vi "Process.vi"(8 "error in":errorcluster, 11 "Example Instrument UI":refnum<class "Instrument UI.Framework-Template.lvclass">) -> (0 "error out":errorcluster, 3 "Example Instrument UI out":refnum<class "Instrument UI.Framework-Template.lvclass">)   [LabVIEW 2019, in "Instrument UI.Framework-Template.lvclass"]
doc: "---------------------------------------------------------------\nJKI State Machine Objects™\nhttp://jki.net/state-machine-objects/\nCopyright (C) 2005-2015, JKI <info@jki.net>\nALL RIGHTS RESERVEDJKI State Machine Objects (SMO) 1.0.0.5\nJKI - JKI\nCopyright (c) 2016, JKI"
uses:
  Instrument UI.Framework-Template.lvclass
  C:/Program Files (x86)/National Instruments/LabVIEW 2019/vi.lib/JKI/JKI SMO/SMO/SMO.lvclass
  C:/Users/patrick/Documents/GitHub/Instrument-Framework/lvsrc/SMOs/Instrument UI/Instrument UI.lvclass
  C:/Program Files (x86)/National Instruments/LabVIEW 2019/vi.lib/JKI/JKI SMO/SMO.UI/SMO.UI.lvclass
  Instrument.Framework-Template/Typedefs/Instrument.Framework-Template.getAll--Cluster.ctl
  Instrument.Framework-Template/Instrument.Framework-Template.lvclass
  C:/Users/patrick/Documents/GitHub/Instrument-Framework/lvsrc/SMOs/Instrument/Instrument.lvclass
  Instrument UI.Framework-Template.UI--Cluster.ctl
  Instrument.Framework-Template/Typedefs/Instrument.Framework-Template.Configuration--Cluster.ctl
  SMOs/Configuration/Configuration.lvclass
  SMOs/Instrument UI/Instrument UI.lvclass/Instrument UI.ctl
  <vilib>/JKI/JKI SMO/SMO/SMO.lvclass/SMO.ctl
  SMOs/Configuration/Configuration.lvclass/Configuration.ctl
  SMOs/Instrument/Instrument.lvclass/Instrument.ctl
  SMOs/Instrument/Typedefs/Client Type--Enum.ctl
  614f1787-3484-4d72-b522-1f8c221dac07.vi
  064e3a37-d4cf-416d-9c97-81a00de9d50c.vi
  <vilib>/JKI/JKI SMO/SMO/Private/ReftoDVR--SMO.vi
  614f1787-3484-4d72-b522-1f8c221dac07.vi/6126265b-52a9-4036-b9ab-d7def26448fd.vi
  064e3a37-d4cf-416d-9c97-81a00de9d50c.vi/2934c5b6-9d9a-4612-aef0-474eff5135e3.vi
  614f1787-3484-4d72-b522-1f8c221dac07.vi/6126265b-52a9-4036-b9ab-d7def26448fd.vi/3777206e-62d3-4194-bbb6-d708f28c6636.vi
  SMOs/Instrument/API/Send and Receive.vi
  614f1787-3484-4d72-b522-1f8c221dac07.vi/6126265b-52a9-4036-b9ab-d7def26448fd.vi/c2acc09a-a3b2-411f-96f0-93bdcc04d904.vi
  SMOs/Instrument/Private/Get Client Type.vi
  064e3a37-d4cf-416d-9c97-81a00de9d50c.vi/2934c5b6-9d9a-4612-aef0-474eff5135e3.vi/d31bd197-f2cf-45ec-b348-66ecc1fb7fa3.vi
  064e3a37-d4cf-416d-9c97-81a00de9d50c.vi/2934c5b6-9d9a-4612-aef0-474eff5135e3.vi/bcf0d896-5092-4459-a902-822cb84f3d2f.vi
  614f1787-3484-4d72-b522-1f8c221dac07.vi/6126265b-52a9-4036-b9ab-d7def26448fd.vi/3777206e-62d3-4194-bbb6-d708f28c6636.vi/a171245e-ace2-4a31-ad0e-c1ba96aac09f.vi
  614f1787-3484-4d72-b522-1f8c221dac07.vi/6126265b-52a9-4036-b9ab-d7def26448fd.vi/3777206e-62d3-4194-bbb6-d708f28c6636.vi/314606e5-fab2-4c4b-855f-38e561406072.vi
  614f1787-3484-4d72-b522-1f8c221dac07.vi/6126265b-52a9-4036-b9ab-d7def26448fd.vi/c2acc09a-a3b2-411f-96f0-93bdcc04d904.vi/068c89fb-261c-4114-b3e0-8879b2039521.vi
  614f1787-3484-4d72-b522-1f8c221dac07.vi/6126265b-52a9-4036-b9ab-d7def26448fd.vi/c2acc09a-a3b2-411f-96f0-93bdcc04d904.vi/70e8e4d8-081c-4447-abab-7ffc08a24431.vi
  064e3a37-d4cf-416d-9c97-81a00de9d50c.vi/2934c5b6-9d9a-4612-aef0-474eff5135e3.vi/d31bd197-f2cf-45ec-b348-66ecc1fb7fa3.vi/16df6886-ccac-4f12-823d-852507d7b6d3.vi
  064e3a37-d4cf-416d-9c97-81a00de9d50c.vi/2934c5b6-9d9a-4612-aef0-474eff5135e3.vi/d31bd197-f2cf-45ec-b348-66ecc1fb7fa3.vi/d363edf0-f48d-4095-b52d-a98fc5c23e31.vi
  064e3a37-d4cf-416d-9c97-81a00de9d50c.vi/2934c5b6-9d9a-4612-aef0-474eff5135e3.vi/bcf0d896-5092-4459-a902-822cb84f3d2f.vi/3efd9854-12da-426d-b303-5f5dfdd99cd3.vi
  064e3a37-d4cf-416d-9c97-81a00de9d50c.vi/2934c5b6-9d9a-4612-aef0-474eff5135e3.vi/bcf0d896-5092-4459-a902-822cb84f3d2f.vi/021688bb-175a-4f04-92c2-7b75fc3f16e3.vi
  614f1787-3484-4d72-b522-1f8c221dac07.vi/6126265b-52a9-4036-b9ab-d7def26448fd.vi/c2acc09a-a3b2-411f-96f0-93bdcc04d904.vi/068c89fb-261c-4114-b3e0-8879b2039521.vi/f4340ad4-3f7d-43fc-a5b8-8cfecf0320e0.vi
  614f1787-3484-4d72-b522-1f8c221dac07.vi/6126265b-52a9-4036-b9ab-d7def26448fd.vi/c2acc09a-a3b2-411f-96f0-93bdcc04d904.vi/068c89fb-261c-4114-b3e0-8879b2039521.vi/09137493-ac28-451c-9813-f227a1b20a03.vi
  064e3a37-d4cf-416d-9c97-81a00de9d50c.vi/2934c5b6-9d9a-4612-aef0-474eff5135e3.vi/bcf0d896-5092-4459-a902-822cb84f3d2f.vi/3efd9854-12da-426d-b303-5f5dfdd99cd3.vi/ec8d0cc2-9f9f-4698-9277-550a01addf9f.vi
  064e3a37-d4cf-416d-9c97-81a00de9d50c.vi/2934c5b6-9d9a-4612-aef0-474eff5135e3.vi/bcf0d896-5092-4459-a902-822cb84f3d2f.vi/3efd9854-12da-426d-b303-5f5dfdd99cd3.vi/599ad89e-f603-4806-a637-659fe558540e.vi
  SMOs/Instrument/Private/Get RC Connection Status.vi
  SMOs/Instrument/API/Enum to String.vi
  SMOs/RemoteControl/API/Send and Receive.vi
  <vilib>/Utility/Data Type/Get Type Information.vi
  <vilib>/JDP Science/JSONtext/JSON text to Variant.vi
  <vilib>/JDP Science/JSONtext/Variant to JSON Text.vi
  <vilib>/National Instruments/GUID Generator/Guid Generator.vi
  SMOs/Instrument/Private/Instrument.MessageFromProcess.EventStructure.vi
  SMOs/Instrument/Instrument.lvclass
  <vilib>/JDP Science/JSONtext/LVClass Serializer/JSONtext LVClass Serializer.lvclass
  SMOs/Instrument UI/Instrument UI.lvclass
  <vilib>/JKI/JKI SMO/SMO/SMO.lvclass
  <vilib>/JKI/JKI SMO/SMO.UI/SMO.UI.lvclass
panel:
  in  "Parameter 2":string
  out "Numeric":u32
  in  "Set Parameter":bool
  in  "Parameter":dbl
  in  "STOP":bool
  out "SMO string":string
  out "SMO Boolean":bool
  out "Logger SMO":dbl
  out "Levy 1":dbl
  # "#todo\nmake UI here. maybe include a nice picture of the hardware?"
  # "#todo\nadd buttons to do stuff (e.g., change a setting)\nButtons should trigger an event"
  # "#todo\nresize this box if you want your UI to be different size"
  # "SMO UI Template"
  # "For instructions on how to use the JKI State Machine Objects, examples and video tutorials, visit:\nhttp://jki.net/state-machine-objects/\n\nJKI State Machine Objects™\nhttp://jki.net/state-machine-objects/\nCopyright (C) 2005-2015, JKI <info@jki.net>\nALL RIGHTS RESERVED"
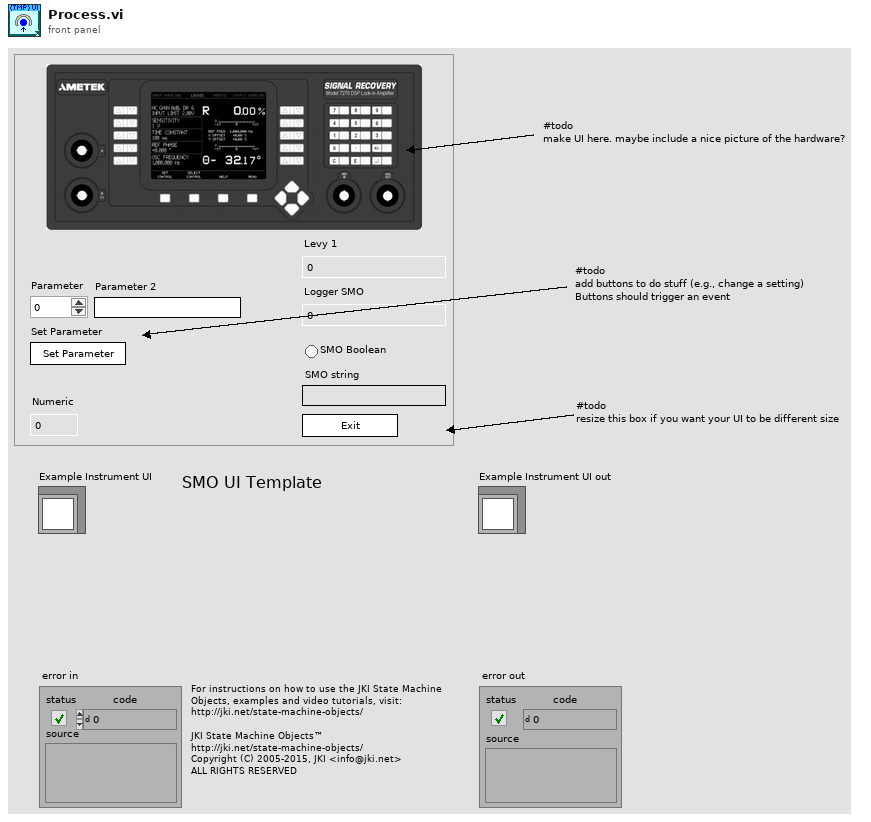
[diagram p1: front panel]
types:
  T1 = enum32{"invalid app kind", "Development System", "Run Time System", "Student Edition", "Embedded LabVIEW", "Evaluation", "Custom"}
  T2 = enum32{"Invalid", "Standard", "Closed", "Hidden", "Minimized", "Maximized"}
  T3 = typedef "Instrument.lvclass/Client Type--Enum.ctl" = enum16{"Remote", "Local"}
  T4 = typedef "Instrument.Framework-Template.lvclass/Instrument.Framework-Template.Configuration--Cluster.ctl" = cluster{"Example Setting 1":dbl, "Example Setting 2":dbl, "Example Setting 3":string}
  T5 = typedef "Instrument.Framework-Template.lvclass/Instrument.Framework-Template.getAll--Cluster.ctl" = cluster{"Levy 1":dbl, "Logger SMO":dbl, "SMO Boolean":bool, "SMO String":string}
  T6 = typedef "Instrument UI.Framework-Template.lvclass/Instrument UI.Framework-Template.UI--Cluster.ctl" = cluster{"Parameter":dbl, "Parameter 2":string}
  T7 = cluster{"Core":cluster{"Current VI Reference":refnum<vi>, "Close Panel on Exit?":bool, "error":errorcluster}, "Instrument UI":refnum<class "Instrument UI.Framework-Template.lvclass">, "Instrument":refnum<class "Instrument.Framework-Template.lvclass">, "Configuration":refnum<class "Configuration.lvclass">, "Config Cluster":T4, "getAll":T5, "UI Cluster":T6}
  T8 = cluster{"Current VI Reference":refnum<vi>, "Close Panel on Exit?":bool, "error":errorcluster}
  T9 = typedef "SMO.lvclass/Protected Events.ctl" = cluster{"StopProcesses":refnum<user-event>, "AbortProcesses":refnum<user-event>, "Config Changed":refnum<user-event>, "Dependency":refnum<user-event>}
  T10 = typedef "Instrument.lvclass/PublicEvents--Cluster.ctl" = cluster{"MessageFromProcess":refnum<user-event>}
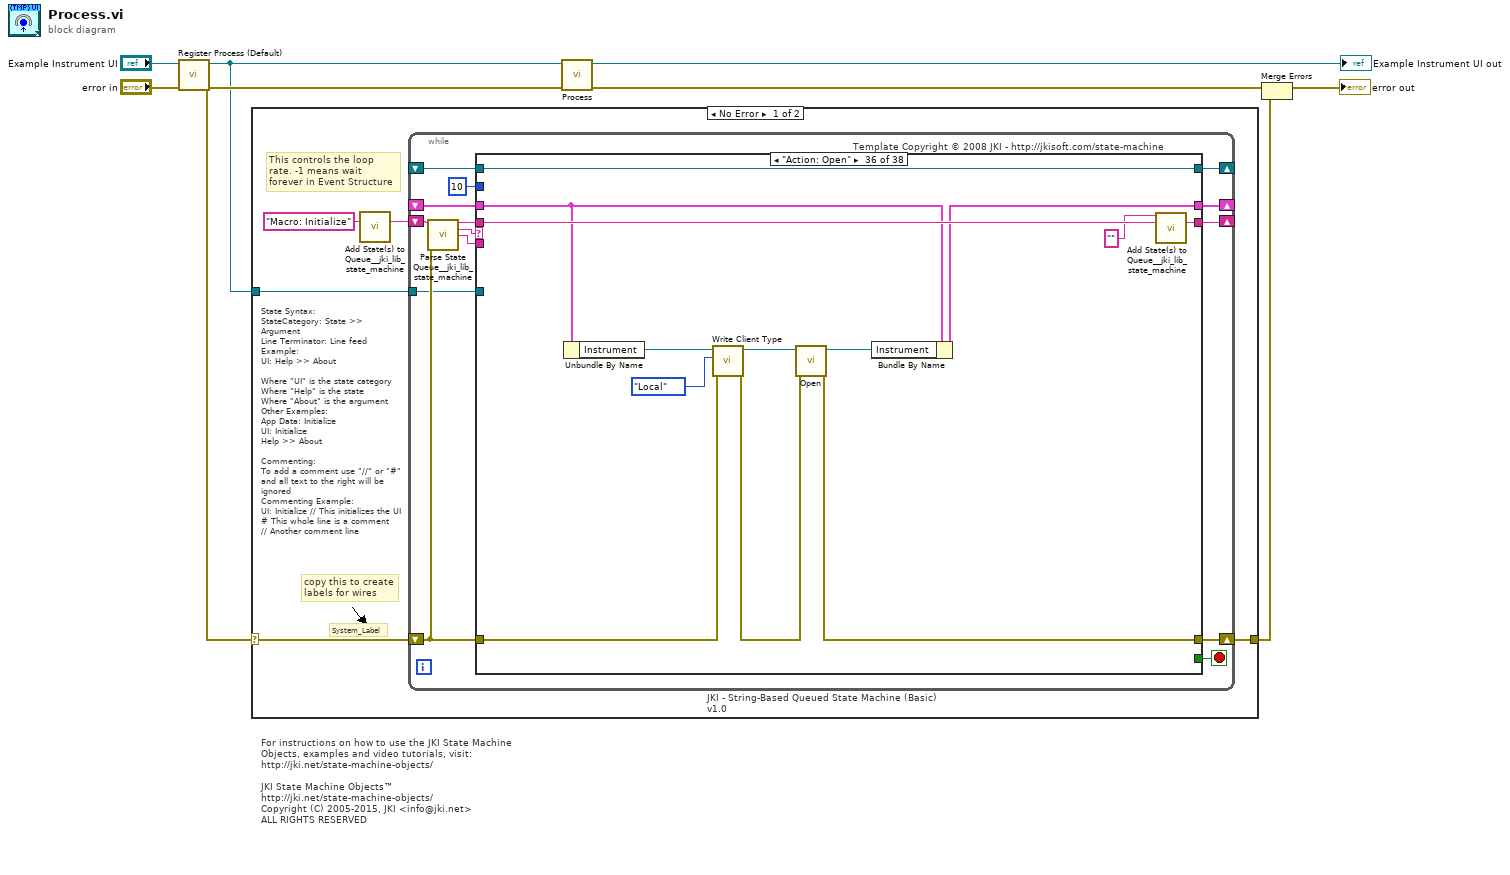
[diagram p0: block diagram]
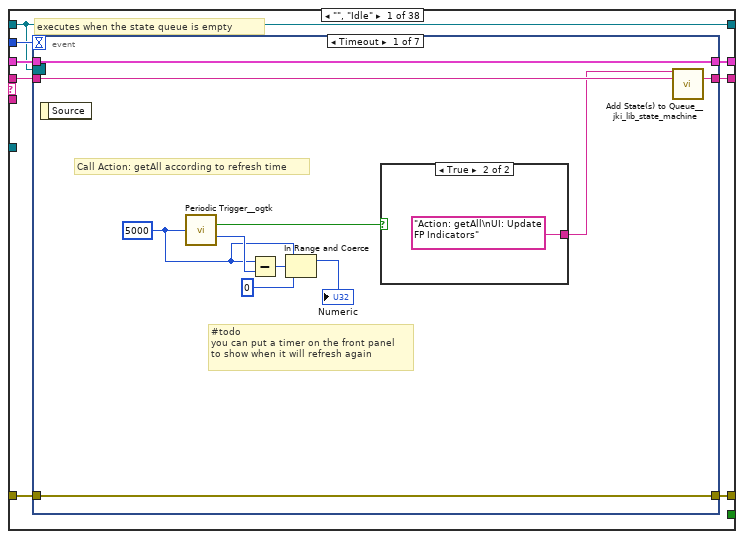
[diagram p2: hidden frame]
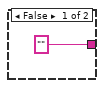
[diagram p3: hidden frame]
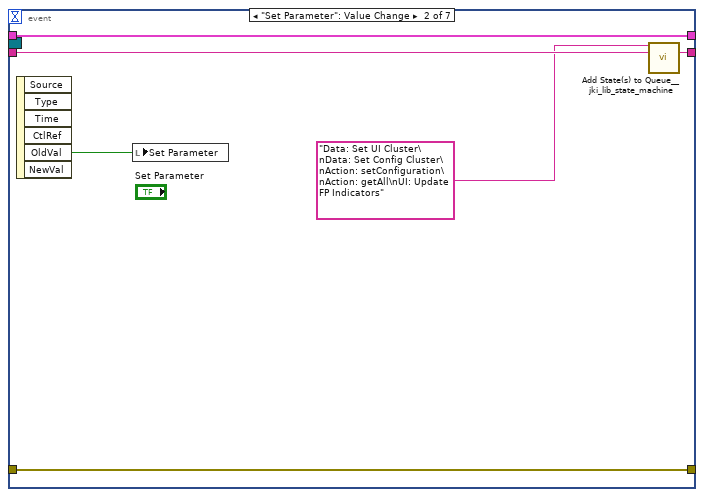
[diagram p4: hidden frame]
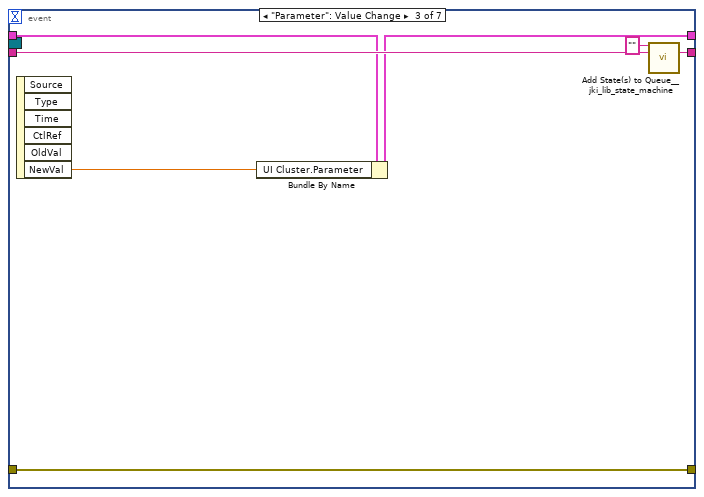
[diagram p5: hidden frame]
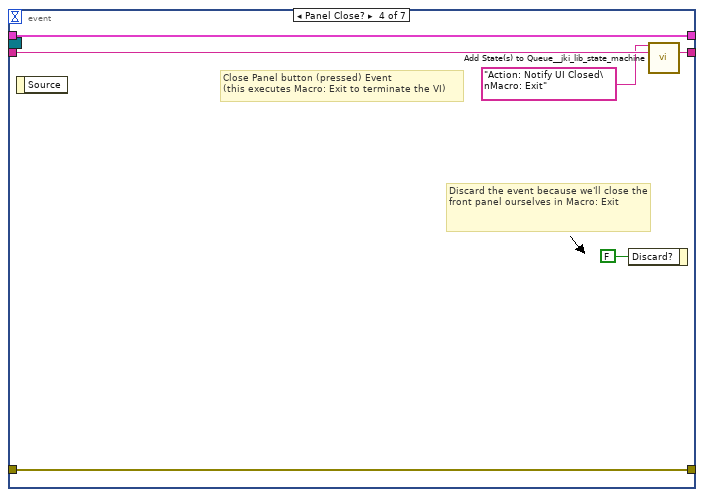
[diagram p6: hidden frame]
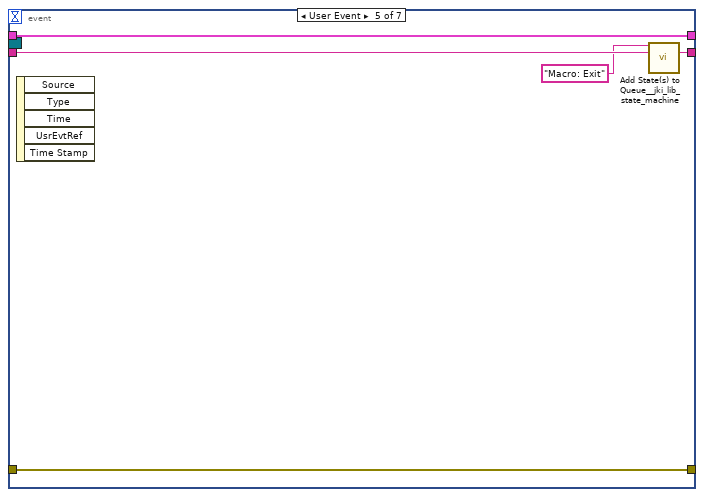
[diagram p7: hidden frame]
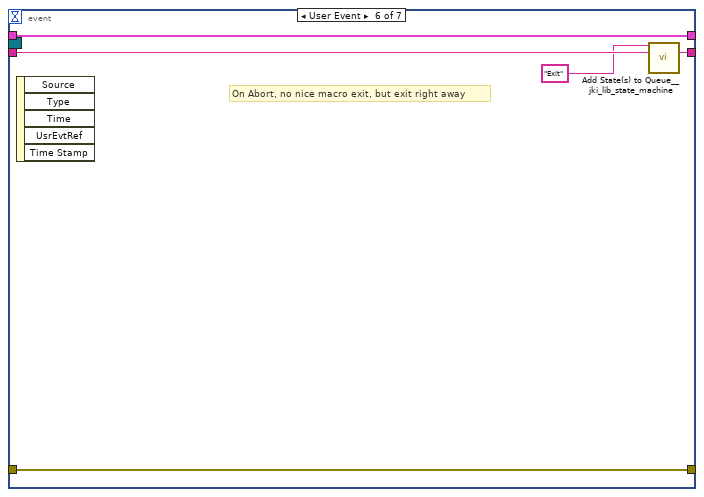
[diagram p8: hidden frame]
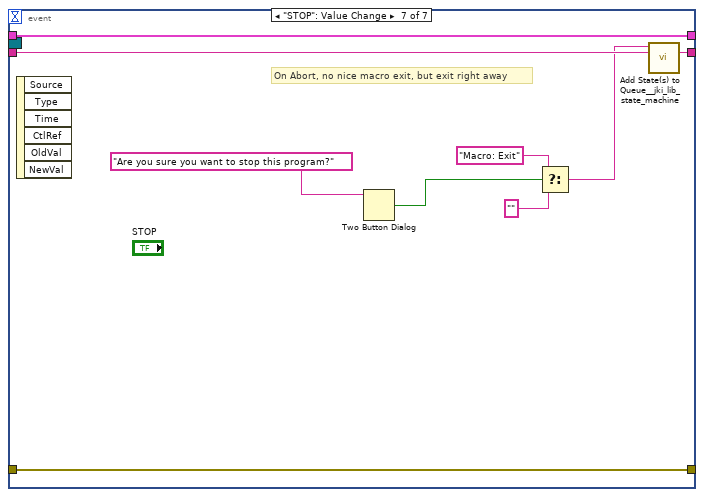
[diagram p9: hidden frame]
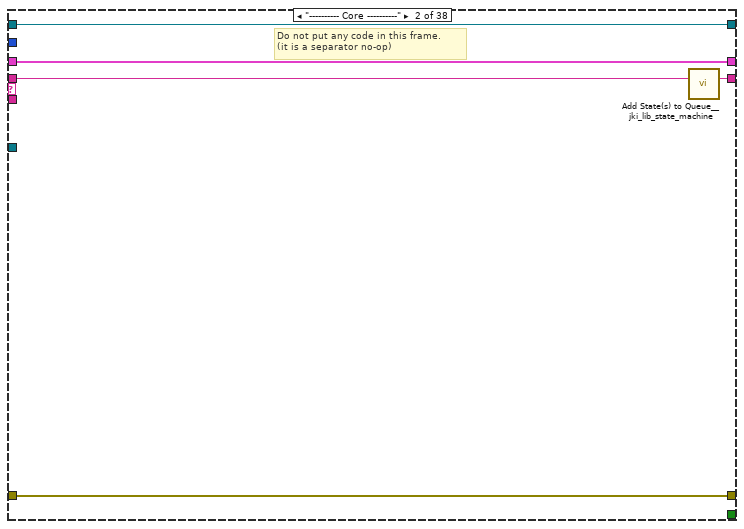
[diagram p10: hidden frame]
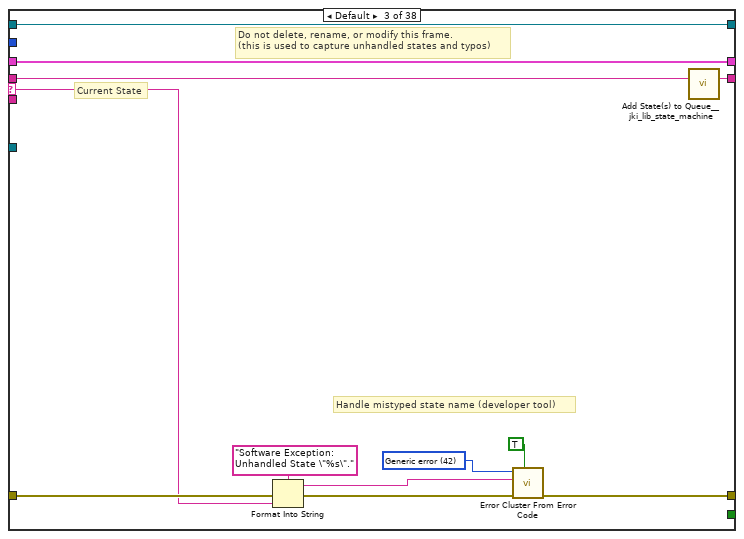
[diagram p11: hidden frame]
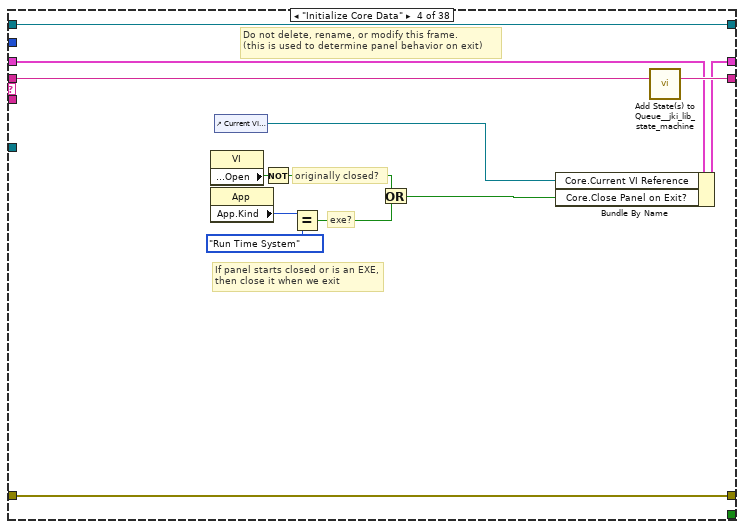
[diagram p12: hidden frame]
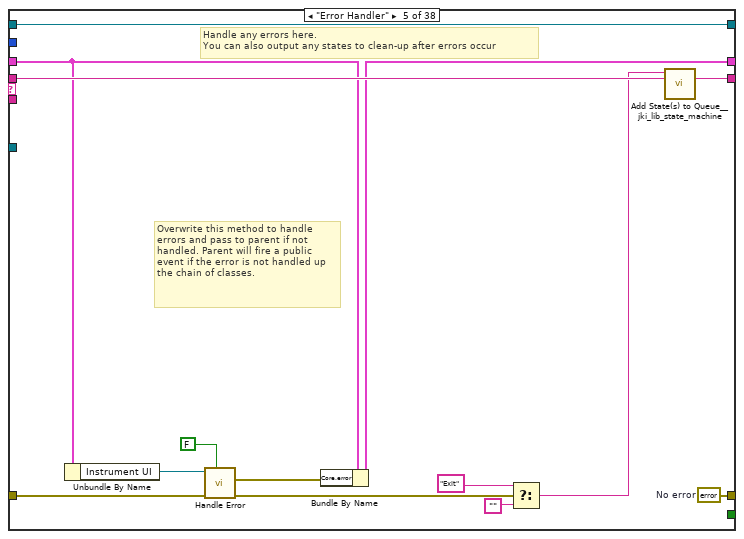
[diagram p13: hidden frame]
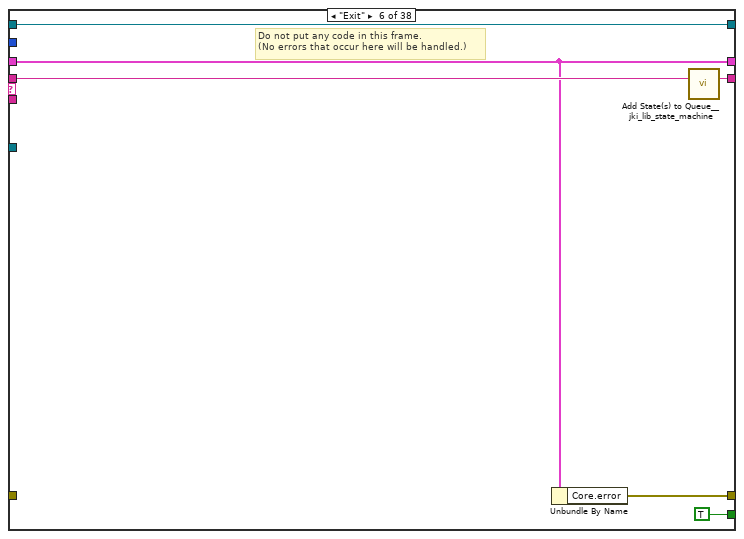
[diagram p14: hidden frame]
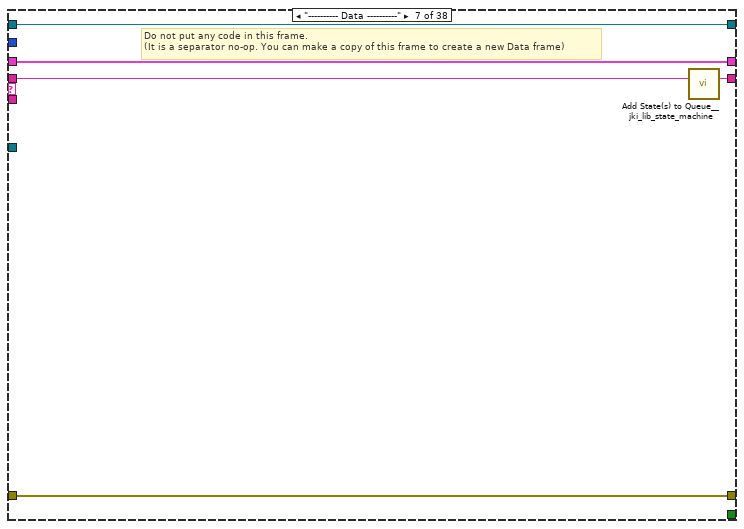
[diagram p15: hidden frame]
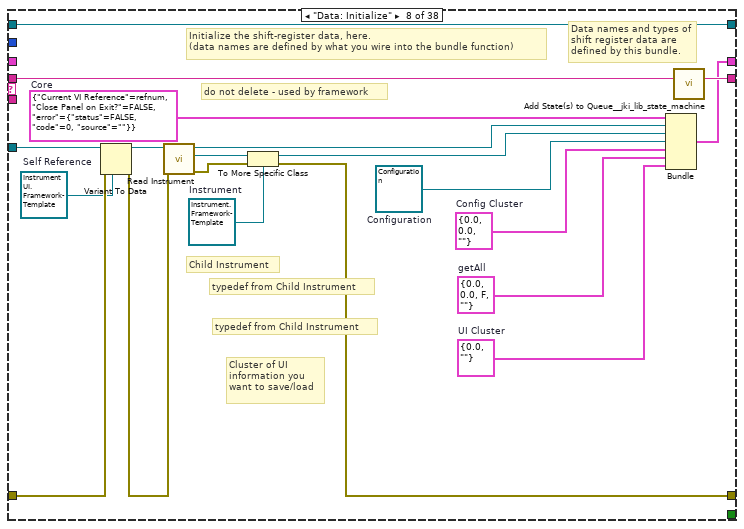
[diagram p16: hidden frame]
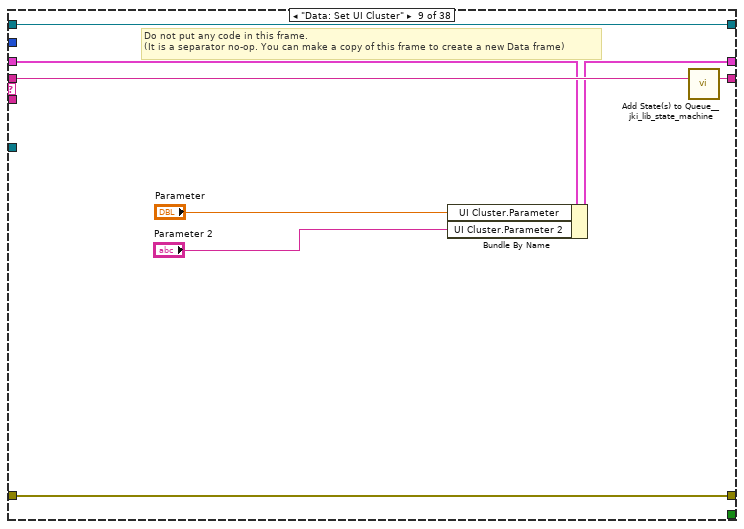
[diagram p17: hidden frame]
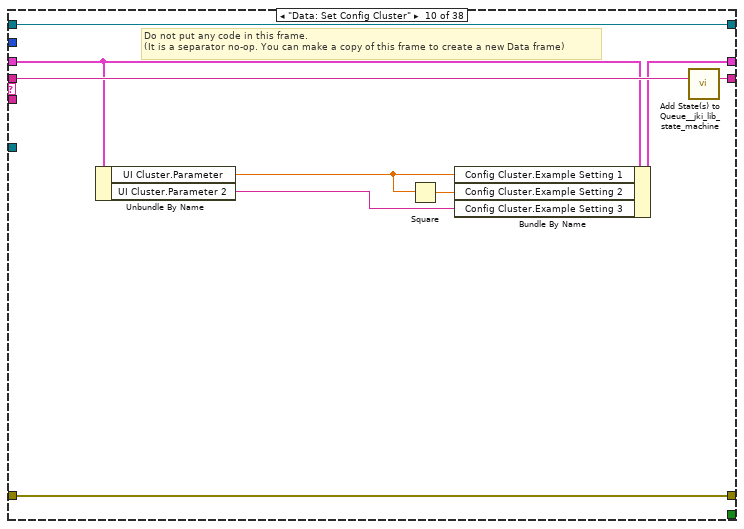
[diagram p18: hidden frame]
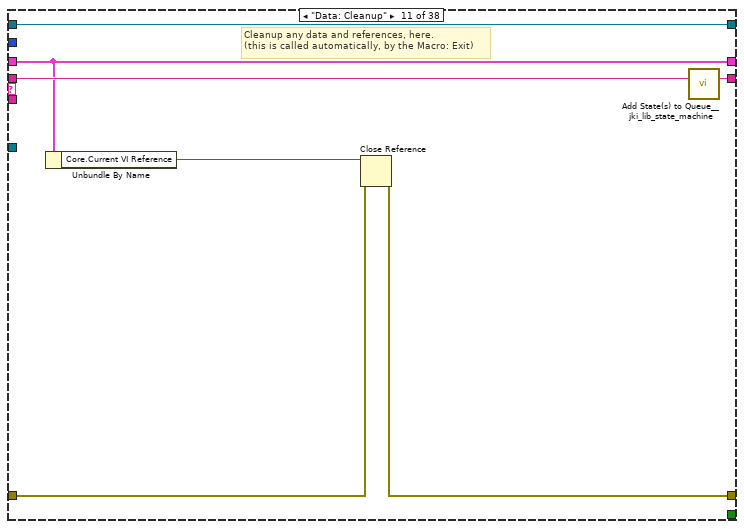
[diagram p19: hidden frame]
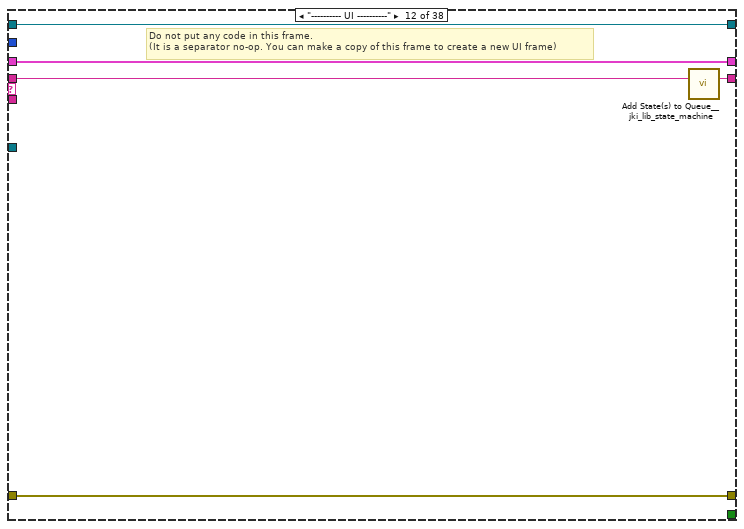
[diagram p20: hidden frame]
diagram:
  # "For instructions on how to use the JKI State Machine Objects, examples and video tutorials, visit:\nhttp://jki.net/state-machine-objects/\n\nJKI State Machine Objects™\nhttp://jki.net/state-machine-objects/\nCopyright (C) 2005-2015, JKI <info@jki.net>\nALL RIGHTS RESERVED"
  n1 = call <vilib>:"Register Process (Default).vi"("error in (no error)"="error in", "SMO"="Example Instrument UI") -> ("error out"=w5:errorcluster, "SelfRef"=w4:refnum<class "Instrument UI.Framework-Template.lvclass">)  [unwired: 8 in]
  n2 = case shown="No Error" w5 {
    selector: w5 -> [w10 w453]
    tunnel: w4 -> [w11 _]
    tunnel: [w9 w453] -> w1
    frame No Error {
      # "State Syntax:\nStateCategory: State >> Argument\nLine Terminator: Line feed\nExample:\nUI: Help >> About\n\nWhere \"UI\" is the state category\nWhere \"Help\" is the state\nWhere \"About\" is the argument\nOther Examples:\nApp Data: Initialize\nUI: Initialize\nHelp >> About\n\nCommenting:\nTo add a comment use \"//\" or \"#\" and all text to the right will be ignored\nCommenting Example:\nUI: Initialize // This initializes the UI\n# This whole line is a comment\n// Another comment line"
      # "copy this to create labels for wires"
      # "This controls the loop rate. -1 means wait forever in Event Structure"
      # "System_Label"
      n3 = call <vilib>:"Add State(s) to Queue__jki_lib_state_machine.vi"("State(s) in (\"\")"="Macro: Initialize") -> ("States Out"=w13:string)  [unwired: 14 in]
      n4 = while "JKI - String-Based Queued State Machine (Basic) v1.0" {
        shift-right: [w20] -> _
        shift-left: _ -> [w19]
        shift-right: [w23] -> w9
        shift-left: w10 -> [w17]
        shift-right: [w22] -> _
        shift-left: w13 -> [w24]
        tunnel: w11 -> [w16]
        shift-right: [w15] -> _
        shift-left: _ -> [w14]
        stop <- w21 stop-if-true
        # "Template Copyright © 2008 JKI - http://jkisoft.com/state-machine"
        n5 = call <vilib>:"Parse State Queue__jki_lib_state_machine.vi"("State Queue"=w24, "Error In (no error)"=w17) -> ("Remaining States"=w26:string, "Current State"=w27:string, "Arguments"=w25:string)  [unwired: 11 in]
        n6 = case shown="\"Action: Open\"" w27 {
          selector: w27 -> [_ _ w93 _ _ _ _ _ _ _ _ _ _ _ _ _ _ _ _ _ _ _ _ _ _ _ _ _ _ _ _ _ _ _ _ _ _ _]
          tunnel: w26 -> [w35 w91 w97 w116 w130 w136 w141 w161 w169 w178 w185 w190 w197 w204 w214 w221 w237 w269 w278 w284 w290 w305 w310 w321 w328 w333 w346 w352 w357 w372 w380 w392 w399 w406 w418 w431 w441 w452]
          tunnel: w25 -> [_ _ _ _ _ _ _ _ _ _ _ _ _ _ _ w215 w231 _ _ _ _ _ _ _ _ _ _ _ _ _ _ _ _ _ _ _ _ _]
          tunnel: w19 -> [w33 w88 w95 w107 w119 w132 w138 _ w165 w174 w179 w187 w195 w200 w205 w219 w233 w266 w274 w281 w287 w292 w307 w318 w323 w330 w344 w350 w354 w365 w377 w383 w395 w400 w410 w425 w433 w444]
          tunnel: [w32 w89 w99 w113 w121 w131 w139 w143 w167 w176 w181 w188 w192 w202 w206 w216 w234 w267 w276 w282 w288 w303 w308 w312 w324 w331 w339 w347 w355 w358 w375 w384 w396 w401 w415 w428 w438 w449] -> w23
          tunnel: w17 -> [w31 w89 w98 w113 w126 _ w139 w158 w167 w176 w182 w188 w193 w202 w206 w217 w235 w267 w276 w282 w288 w303 w308 w313 w325 w331 w341 w348 w355 w367 w373 w385 w396 w402 w411 w420 w434 w445]
          tunnel: [w34 w90 w96 w115 w129 w135 w140 w160 w168 w177 w184 w189 w196 w203 w213 w220 w236 w268 w277 w283 w289 w304 w309 w320 w327 w332 w345 w351 w356 w371 w379 w391 w398 w405 w417 w430 w440 w451] -> w22
          tunnel: [_ _ _ _ _ TRUE _ _ _ _ _ _ _ _ _ _ _ _ _ _ _ _ _ _ _ _ _ _ _ _ _ _ _ _ _ _ _ _] -> w21
          tunnel: [w30 w88 w95 w114 w118 w132 w138 w159 w164 w173 w179 w187 w195 w200 w205 w219 w233 w266 w274 w281 w287 w292 w307 w318 w323 w330 w344 w350 w354 w369 w377 w381 w394 w400 w412 w426 w435 w446] -> w20
          tunnel: 10 ("Timeout") -> [w29 _ _ _ _ _ _ _ _ _ _ _ _ _ _ _ _ _ _ _ _ _ _ _ _ _ _ _ _ _ _ _ _ _ _ _ _ _]
          tunnel: w16 -> [_ _ _ _ _ _ _ w156 _ _ _ _ _ _ _ _ _ _ _ _ _ _ _ _ _ _ _ _ _ _ _ _ _ _ _ _ _ _]
          tunnel: [w28 w87 w92 w104 w128 w133 w137 w155 w166 w175 w180 w186 w194 w201 w212 w218 w230 w265 w275 w280 w286 w297 w306 w319 w326 w329 w343 w349 w353 w370 w378 w390 w397 w404 w416 w429 w439 w450] -> w15
          tunnel: w14 -> [w28 w87 w92 w104 w128 w133 w137 w155 w166 w175 w180 w186 w194 w201 w212 w218 w230 w265 w275 w280 w286 w297 w306 w319 w326 w329 _ w349 w353 w370 w378 w390 w397 w404 w416 w429 w439 w450]
          frame "", "Idle" {
            # "executes when the state queue is empty"
            n7 = event shown="[0] Timeout" {
              selector: w28 -> [_ _ _ _ _ _ _]
              dyn-events: _ -> [_ _ _ _ _ _ _]
              timeout: w29 -> [_ _ _ _ _ _ _]
              tunnel: w35 -> [w46 w54 w61 w67 w72 w77 w86]
              tunnel: [w45 w53 w60 w66 w71 w76 w85] -> w34
              tunnel: w33 -> [w43 w51 w57 w63 w69 w74 w83]
              tunnel: [w44 w52 w59 w62 w70 w75 w84] -> w32
              tunnel: w31 -> [w44 w52 w59 w62 w70 w75 w84]
              tunnel: [w43 w51 w56 w63 w69 w74 w83] -> w30
              event Timeout {
                w37 = u32 5000 ("time (ms)")
                # "#todo\nyou can put a timer on the front panel\nto show when it will refresh again"
                # "Call Action: getAll according to refresh time"
                n8 = event-data() -> ()  [unwired: 1 in, 1 out]
                n9 = call <userlib>:"Periodic Trigger__ogtk.vi"("time (ms)"=w37) -> ("Triggered"=w41:bool, "timer value"=w40:u32)  [unwired: 12 in, 1 out]
                n10 = Subtract(x=w37, y=w40) -> (x-y=w39:u32)
                n11 = In Range and Coerce(upper limit=w37, x=w39, lower limit=u32 0) -> (coerced(x)=→"Numeric":u32)  [unwired: 1 out]
                n12 = case shown="True" w41 {
                  tunnel: ["" ("State(s) in Front (\"\")") "Action: getAll\nUI: Update FP Indicators" ("State(s) in Front (\"\")")] -> w42
                  frame False {
                  }
                  frame True {
                  }
                }
                n13 = call <vilib>:"Add State(s) to Queue__jki_lib_state_machine.vi"("State(s) in Front (\"\")"=w42, "State(s) in (\"\")"=w46) -> ("States Out"=w45:string)  [unwired: 13 in]
              }
              event "Set Parameter": Value Change {
                n14 = event-data() -> ("OldVal"=w50:bool)  [unwired: 1 in, 5 out]
                n15 = local write "Set Parameter"(w50) -> ()
                n16 = call <vilib>:"Add State(s) to Queue__jki_lib_state_machine.vi"("State(s) in Front (\"\")"="Data: Set UI Cluster\nData: Set Config Cluster\nAction: setConfiguration\nAction: getAll\nUI: Update FP Indicators" ("State(s) in Front (\"\")"), "State(s) in (\"\")"=w54) -> ("States Out"=w53:string)  [unwired: 13 in]
              }
              event "Parameter": Value Change {
                n17 = event-data() -> ("NewVal"=w58:dbl)  [unwired: 1 in, 5 out]
                n18 = Bundle By Name(cluster=w57, "UI Cluster.Parameter"=w58) -> (w56:T7)
                n19 = call <vilib>:"Add State(s) to Queue__jki_lib_state_machine.vi"("State(s) in Front (\"\")"="" ("State(s) in Front (\"\")"), "State(s) in (\"\")"=w61) -> ("States Out"=w60:string)  [unwired: 13 in]
              }
              event Panel Close? {
                # "Discard the event because we'll close the front panel ourselves in Macro: Exit"
                # "Close Panel button (pressed) Event\n(this executes Macro: Exit to terminate the VI)"
                n20 = event-data() -> ()  [unwired: 1 in, 1 out]
                n21 = event-data("Discard?"=FALSE) -> ()  [unwired: 1 in, 1 out]
                n22 = call <vilib>:"Add State(s) to Queue__jki_lib_state_machine.vi"("State(s) in Front (\"\")"="Action: Notify UI Closed\nMacro: Exit", "State(s) in (\"\")"=w67) -> ("States Out"=w66:string)  [unwired: 13 in]
              }
              event User Event {
                n23 = event-data() -> ()  [unwired: 1 in, 5 out]
                n24 = call <vilib>:"Add State(s) to Queue__jki_lib_state_machine.vi"("State(s) in Front (\"\")"="Macro: Exit", "State(s) in (\"\")"=w72) -> ("States Out"=w71:string)  [unwired: 13 in]
              }
              event User Event {
                # "On Abort, no nice macro exit, but exit right away"
                n25 = event-data() -> ()  [unwired: 1 in, 5 out]
                n26 = call <vilib>:"Add State(s) to Queue__jki_lib_state_machine.vi"("State(s) in Front (\"\")"="Exit", "State(s) in (\"\")"=w77) -> ("States Out"=w76:string)  [unwired: 13 in]
              }
              event "STOP": Value Change {
                # "On Abort, no nice macro exit, but exit right away"
                n27 = event-data() -> ()  [unwired: 1 in, 6 out]
                n28 = Two Button Dialog(message="Are you sure you want to stop this program?") -> (T button?=w82:bool)  [unwired: 2 in]
                n29 = Select(t="Macro: Exit", s=w82, f="") -> (s? t:f=w78:string)
                n30 = call <vilib>:"Add State(s) to Queue__jki_lib_state_machine.vi"("State(s) in Front (\"\")"=w78, "State(s) in (\"\")"=w86) -> ("States Out"=w85:string)  [unwired: 13 in]
              }
            }
          }
          frame "---------- Core ----------" {
            # "Do not put any code in this frame.\n(it is a separator no-op)"
            n31 = call <vilib>:"Add State(s) to Queue__jki_lib_state_machine.vi"("State(s) in (\"\")"=w91) -> ("States Out"=w90:string)  [unwired: 14 in]
          }
          frame Default {
            w102 = 42 items=["No error", "Argument error", "Memory is full", "Out of zone", "End of file", "File already open", "Generic file I/O error", "File not found", "File permission error", "Disk is full", "Duplicate path", "Too many files open", "System feature not enabled", "Resource file not found", "Cannot add resource", "Resource not found", "Image not found", "Image memory error", "Pen does not exist", "Config type invalid", "Config token not found", "Config parse error", "Config memory error", "Bad external code format", "Bad external code offset", "External code not present", "Null window", "Destroy window error", "Null menu", "Print aborted", "Bad print record", "Print driver error", "Windows error during printing", "Memory error during printing", "Print dialog error", "Generic print error", "Invalid device refnum", "Device not found", "Device parameter error", "Device unit error", "Cannot open device", "Device call aborted", "Generic error", "Cancelled by user", "Object ID too low", "Object ID too high", "Object not in heap", "Unknown heap", "Unknown object (invalid DefProc)", "Unknown object (DefProc not in table)", "Message out of range", "Invalid (null) method", "Unknown message", "Manager call not supported", "Bad address", "Network operation in progress", "Network operation timed out", "Connection is busy", "Network attribute not supported", "Network error", "Address in use", "System out of memory", "Connection aborted", "Connection refused", "Not connected", "Already connected", "Connection closed", "Initialization error (interapplication manager)", "Bad occurrence", "Wait on unbound occurrence handler", "Occurrence queue overflow", "Datalog type conflict", "Unused", "Unrecognized type (interapplication manager)", "Memory corrupt", "Failed to make temporary DLL", "Old CIN version", "Drag socket not found", "Failed to load drop-object", "Failed to register OLE object", "Failed to release OLE object", "Format specifier type mismatch", "Unknown format specifier", "Too few format specifiers", "Too many format specifiers", "Scan failed", "Newer CIN version", "Error converting to variant", "Runtime menu error", "Password tampered", "Variant attribute not found", "Incompatible variant data type", "Event data is not available", "Event Store is not present", "Occurrence is not found", "Event Queue is not created", "Event info is not available", "Refnum passed is NULL", "Error retrieving Class GUID", "Error retrieving CoClass GUID", "Error retrieving TypeLib GUID.", "Bad built application magic bytes.", "Specific driver is different from the specific driver associated with the Logical Name.", "There is no session opened to the class driver.", "Max Error", "MAX - Error with config objects", "MAX - Error loading configuration", "MAX - Group not supported"]
            # "Current State"
            # "Do not delete, rename, or modify this frame.\n(this is used to capture unhandled states and typos)"
            # "Handle mistyped state name (developer tool)"
            n32 = Format Into String(format string="Software Exception: Unhandled State \"%s\"." ("message"), error in=w98, w93) -> (resulting string=w101:string, error out=w100:errorcluster)  [unwired: 1 in]
            n33 = call <vilib>:"Error Cluster From Error Code.vi"("show call chain? (False)"=TRUE, "error in (no error)"=w100, "error message (\"\")"=w101, "error code (0)"=w102) -> ("error out"=w99:errorcluster)  [unwired: 5 in]
            n34 = call <vilib>:"Add State(s) to Queue__jki_lib_state_machine.vi"("State(s) in (\"\")"=w97) -> ("States Out"=w96:string)  [unwired: 14 in]
          }
          frame "Initialize Core Data" {
            # "Do not delete, rename, or modify this frame.\n(this is used to determine panel behavior on exit)"
            # "originally closed?"
            # "exe?"
            # "If panel starts closed or is an EXE, then close it when we exit"
            n35 = property class="VI"() -> ("Front Panel.Open"=w112:bool)  [unwired: 2 in, 2 out]
            n36 = property class="App"() -> ("App.Kind"=w111:T1)  [unwired: 2 in, 2 out]
            n37 = control-ref of="Current VI Reference"() -> (w105:refnum<vi>)
            n38 = Not(x=w112) -> (.not. x?=w109:bool)
            n39 = Equal?(x=w111, y=T1."Run Time System" ("Application:Kind")) -> (x = y?=w108:bool)
            n40 = Or(x=w109, y=w108) -> (x .or. y?=w106:bool)
            n41 = Bundle By Name(cluster=w107, "Core.Current VI Reference"=w105, "Core.Close Panel on Exit?"=w106) -> (w114:T7)
            n42 = call <vilib>:"Add State(s) to Queue__jki_lib_state_machine.vi"("State(s) in (\"\")"=w116) -> ("States Out"=w115:string)  [unwired: 14 in]
          }
          frame "Error Handler" {
            w121 = errorcluster {"status"=FALSE, "code"=0, "source"=""}  # No error
            # "Overwrite this method to handle errors and pass to parent if not handled. Parent will fire a public event if the error is not handled up the chain of classes."
            # "Handle any errors here.\nYou can also output any states to clean-up after errors occur"
            n43 = Unbundle By Name(w119) -> ("Instrument UI"=w127:refnum<class "Instrument UI.Framework-Template.lvclass">)
            n44 = call-dynamic "Handle Error.vi"("Stop on Unhandled Error (T)"=FALSE, "error in"=w126, "SMO"=w127) -> ("handling error"=w122:errorcluster, "Unhandled error"=w120:errorcluster)  [unwired: 6 in, 1 out]
            n45 = Bundle By Name(cluster=w119, "Core.error"=w120) -> (w118:T7)
            n46 = Select(t="Exit", s=w122, f="") -> (s? t:f=w123:string)
            n47 = call <vilib>:"Add State(s) to Queue__jki_lib_state_machine.vi"("State(s) in Front (\"\")"=w123, "State(s) in (\"\")"=w130) -> ("States Out"=w129:string)  [unwired: 13 in]
          }
          frame "Exit" {
            # "Do not put any code in this frame.\n(No errors that occur here will be handled.)"
            n48 = Unbundle By Name(w132) -> ("Core.error"=w131:errorcluster)
            n49 = call <vilib>:"Add State(s) to Queue__jki_lib_state_machine.vi"("State(s) in (\"\")"=w136) -> ("States Out"=w135:string)  [unwired: 14 in]
          }
          frame "---------- Data ----------" {
            # "Do not put any code in this frame.\n(It is a separator no-op. You can make a copy of this frame to create a new Data frame)"
            n50 = call <vilib>:"Add State(s) to Queue__jki_lib_state_machine.vi"("State(s) in (\"\")"=w141) -> ("States Out"=w140:string)  [unwired: 14 in]
          }
          frame "Data: Initialize" {
            w142 = refnum<class "Configuration.lvclass"> refnum  # Configuration
            w145 = T4 {"Example Setting 1"=0.0, "Example Setting 2"=0.0, "Example Setting 3"=""}  # Config Cluster
            w147 = T6 {"Parameter"=0.0, "Parameter 2"=""}  # UI Cluster
            w149 = refnum<class "Instrument.Framework-Template.lvclass"> refnum  # Instrument
            w153 = T5 {"Levy 1"=0.0, "Logger SMO"=0.0, "SMO Boolean"=FALSE, "SMO String"=""}  # getAll
            w154 = T8 {"Current VI Reference"=refnum, "Close Panel on Exit?"=FALSE, "error"={"status"=FALSE, "code"=0, "source"=""}}  # Core
            w157 = refnum<class "Instrument UI.Framework-Template.lvclass"> refnum  # Self Reference
            # "typedef from Child Instrument"
            # "Cluster of UI\ninformation you\nwant to save/load"
            # "Child Instrument"
            # "typedef from Child Instrument"
            # "do not delete - used by framework"
            # "Data names and types of shift register data are defined by this bundle."
            # "Initialize the shift-register data, here.\n(data names are defined by what you wire into the bundle function)"
            n51 = Variant To Data(error in=w158, type=w157, Variant=w156) -> (data=w151:refnum<class "Instrument UI.Framework-Template.lvclass">, error out=w152:errorcluster)
            n52 = call "Read Instrument.vi"("error in (no error)"=w152, "Instrument UI in"=w151) -> ("error out"=w146:errorcluster, "Instrument"=w148:refnum<class "Instrument.lvclass">, "Instrument UI"=w150:refnum<class "Instrument UI.Framework-Template.lvclass">)  [unwired: 7 in]
            n53 = To More Specific Class(target class=w149, reference=w148, error in=w146) -> (specific class reference=w144:refnum<class "Instrument.Framework-Template.lvclass">, error out=w143:errorcluster)
            n54 = Bundle("Core"=w154, "Instrument UI"=w150, "Instrument"=w144, "Configuration"=w142, "Config Cluster"=w145, "getAll"=w153, "UI Cluster"=w147) -> (w159:T7)  [unwired: 1 in]
            n55 = call <vilib>:"Add State(s) to Queue__jki_lib_state_machine.vi"("State(s) in (\"\")"=w161) -> ("States Out"=w160:string)  [unwired: 14 in]
          }
          frame "Data: Set UI Cluster" {
            # "Do not put any code in this frame.\n(It is a separator no-op. You can make a copy of this frame to create a new Data frame)"
            n56 = Bundle By Name(cluster=w165, "UI Cluster.Parameter"="Parameter", "UI Cluster.Parameter 2"="Parameter 2") -> (w164:T7)
            n57 = call <vilib>:"Add State(s) to Queue__jki_lib_state_machine.vi"("State(s) in (\"\")"=w169) -> ("States Out"=w168:string)  [unwired: 14 in]
          }
          frame "Data: Set Config Cluster" {
            # "Do not put any code in this frame.\n(It is a separator no-op. You can make a copy of this frame to create a new Data frame)"
            n58 = Unbundle By Name(w174) -> ("UI Cluster.Parameter"=w171:dbl, "UI Cluster.Parameter 2"=w172:string)
            n59 = Square(x=w171) -> (x^2=w170:dbl)
            n60 = Bundle By Name(cluster=w174, "Config Cluster.Example Setting 1"=w171, "Config Cluster.Example Setting 2"=w170, "Config Cluster.Example Setting 3"=w172) -> (w173:T7)
            n61 = call <vilib>:"Add State(s) to Queue__jki_lib_state_machine.vi"("State(s) in (\"\")"=w178) -> ("States Out"=w177:string)  [unwired: 14 in]
          }
          frame "Data: Cleanup" {
            # "Cleanup any data and references, here.\n(this is called automatically, by the Macro: Exit)"
            n62 = Unbundle By Name(w179) -> ("Core.Current VI Reference"=w183:refnum<vi>)
            n63 = Close Reference(reference=w183, error in (no error)=w182) -> (error out=w181:errorcluster)
            n64 = call <vilib>:"Add State(s) to Queue__jki_lib_state_machine.vi"("State(s) in (\"\")"=w185) -> ("States Out"=w184:string)  [unwired: 14 in]
          }
          frame "---------- UI ----------" {
            # "Do not put any code in this frame.\n(It is a separator no-op. You can make a copy of this frame to create a new UI frame)"
            n65 = call <vilib>:"Add State(s) to Queue__jki_lib_state_machine.vi"("State(s) in (\"\")"=w190) -> ("States Out"=w189:string)  [unwired: 14 in]
          }
          frame "UI: Initialize" {
            # "size window to decoration box on front panel"
            # "Initialize the User Interface, here.\n(this is called automatically, by the Macro: Init)"
            n66 = invoke on="STOP" class="Bool (strict)" method="Reinit To Default"() -> ()  [unwired: 3 in, 3 out]
            n67 = call <userlib>:"Fit VI window to Largest Dec__ogtk.vi"("error in (no error)"=w193, "border spacing (2 px)"=0) -> ("error out"=w192:errorcluster)  [unwired: 4 in, 1 out]
            n68 = call <vilib>:"Add State(s) to Queue__jki_lib_state_machine.vi"("State(s) in (\"\")"=w197) -> ("States Out"=w196:string)  [unwired: 14 in]
          }
          frame "UI: Update FP Controls" {
            # "Do not put any code in this frame.\n(It is a separator no-op. You can make a copy of this frame to create a new UI frame)"
            n69 = Unbundle By Name(w200) -> ("UI Cluster.Parameter"=w198:dbl, "UI Cluster.Parameter 2"=w199:string)
            n70 = local write "Parameter 2"(w199) -> ()
            n71 = local write "Parameter"(w198) -> ()
            n72 = call <vilib>:"Add State(s) to Queue__jki_lib_state_machine.vi"("State(s) in (\"\")"=w204) -> ("States Out"=w203:string)  [unwired: 14 in]
          }
          frame "UI: Update FP Indicators" {
            # "do this way to have nicer UI or only display what you want"
            n73 = Unbundle By Name(w205) -> ("getAll"=w207:T5)
            n74 = Unbundle By Name(w207) -> ("Levy 1"=→"Levy 1":dbl, "Logger SMO"=→"Logger SMO":dbl, "SMO Boolean"=→"SMO Boolean":bool, "SMO String"=→"SMO string":string)
            n75 = call <vilib>:"Add State(s) to Queue__jki_lib_state_machine.vi"("State(s) in (\"\")"=w214) -> ("States Out"=w213:string)  [unwired: 14 in]
          }
          frame "UI: Cursor Set" {
            # "Argument"
            # "Initialize the User Interface, here.\n(this is called automatically, by the Macro: Init)"
            n76 = disable-structure shown="Default" {
              disable-tunnel: w217 -> [w222 w225]
              disable-tunnel: [w222 w224] -> w216
              disable-tunnel: w215 -> [_ w223]
              frame condition #0 {
              }
              frame condition #1 (active) {
                n77 = case shown="\"Busy\"" w223 {
                  tunnel: w225 -> [w227 w229]
                  tunnel: [w226 w228] -> w224
                  frame "Idle", Default {
                    n78 = call <vilib>:"Unset Busy.vi"("error in (no error)"=w227) -> ("error out"=w226:errorcluster)  [unwired: 10 in]
                  }
                  frame "Busy" {
                    n79 = call <vilib>:"Set Busy.vi"("error in (no error)"=w229) -> ("error out"=w228:errorcluster)  [unwired: 9 in, 1 out]
                  }
                }
              }
            }
            n80 = call <vilib>:"Add State(s) to Queue__jki_lib_state_machine.vi"("State(s) in (\"\")"=w221) -> ("States Out"=w220:string)  [unwired: 14 in]
          }
          frame "UI: Front Panel State" {
            # "Argument"
            # "Set Front Panel Open or Closed\n(Usage: \"UI: Front Panel State >> Open|Close\")"
            n81 = Unbundle By Name(w233) -> ("Core.Current VI Reference"=w232:refnum<vi>)
            n82 = disable-structure shown="Default" {
              disable-tunnel: w235 -> [w241 w264]
              disable-tunnel: [w240 w264] -> w234
              disable-tunnel: w232 -> [w239 _]
              disable-tunnel: w231 -> [w238 _]
              frame condition #0 (active) {
                n83 = case shown="\"Close\"" w238 {
                  tunnel: w241 -> [w245 w258]
                  tunnel: [w247 w259] -> w240
                  tunnel: w239 -> [w246 w256]
                  frame "Open", Default {
                    n84 = property class="VI"(reference=w246, error in=w245) -> (reference out=w243:refnum<vi>, error out=w244:errorcluster, "FP.State"=w242:T2)
                    n85 = case shown="\"Closed\"" w242 {
                      tunnel: [w250 w253] -> w247
                      tunnel: w244 -> [w249 w253]
                      tunnel: w243 -> [w248 _]
                      frame "Closed" {
                        n86 = invoke class="VI" method="FP.Open"(reference=w248, error in=w249, "Activate"=TRUE, "State"=T2."Standard") -> (error out=w250:errorcluster)  [unwired: 1 in, 4 out]
                      }
                      frame Default {
                      }
                    }
                  }
                  frame "Close" {
                    n87 = property class="VI"(reference=w256, error in=w258) -> (reference out=w255:refnum<vi>, error out=w257:errorcluster, "FP.State"=w254:T2)
                    n88 = case shown="Default" w254 {
                      tunnel: [w260 w263] -> w259
                      tunnel: w257 -> [w260 w262]
                      tunnel: w255 -> [_ w261]
                      frame "Invalid", "Closed" {
                      }
                      frame Default {
                        n89 = invoke class="VI" method="FP.Close"(reference=w261, error in=w262) -> (error out=w263:errorcluster)  [unwired: 1 in, 2 out]
                      }
                    }
                  }
                }
              }
              frame condition #1 {
              }
            }
            n90 = call <vilib>:"Add State(s) to Queue__jki_lib_state_machine.vi"("State(s) in (\"\")"=w237) -> ("States Out"=w236:string)  [unwired: 14 in]
          }
          frame "---------- Macro ----------" {
            # "Do not put any code in this frame.\n(It is a separator no-op. You can make a copy of this frame to create a new Macro frame)"
            n91 = call <vilib>:"Add State(s) to Queue__jki_lib_state_machine.vi"("State(s) in (\"\")"=w269) -> ("States Out"=w268:string)  [unwired: 14 in]
          }
          frame "Macro: Initialize" {
            w272 = "UI: Initialize\nMacro: Read UI Config\nAction: Open\n//UI: Front Panel State >> Open"  # UI: Initialize Macro: Read UI Config Action: Open //UI: Front Panel State >> Open
            # "Initialization Macro\n(This is called once, when the VI starts)"
            n92 = call <vilib>:"Add State(s) to Queue__jki_lib_state_machine.vi"("State(s) in Front (\"\")"="Data: Initialize\nInitialize Core Data\nEvents: Register", "State(s) in (\"\")"="Process: Sync", "State(s) at Back (\"\")"=w272) -> ("States Out"=w271:string)  [unwired: 12 in]
            n93 = call <vilib>:"Add State(s) to Queue__jki_lib_state_machine.vi"("State(s) in Front (\"\")"=w271, "State(s) in (\"\")"=w278) -> ("States Out"=w277:string)  [unwired: 13 in]
          }
          frame "Macro: Read UI Config" {
            # "Do not put any code in this frame.\n(It is a separator no-op. You can make a copy of this frame to create a new Macro frame)"
            n94 = call <vilib>:"Add State(s) to Queue__jki_lib_state_machine.vi"("State(s) in Front (\"\")"="Configuration: Initialize\nConfiguration: Read UI Config File\nUI: Update FP Controls" ("State(s) in Front (\"\")"), "State(s) in (\"\")"=w284) -> ("States Out"=w283:string)  [unwired: 13 in]
          }
          frame "Macro: Write UI Config" {
            # "Do not put any code in this frame.\n(It is a separator no-op. You can make a copy of this frame to create a new Macro frame)"
            n95 = call <vilib>:"Add State(s) to Queue__jki_lib_state_machine.vi"("State(s) in Front (\"\")"="Data: Set UI Cluster\nConfiguration: Write UI Config File" ("State(s) in Front (\"\")"), "State(s) in (\"\")"=w290) -> ("States Out"=w289:string)  [unwired: 13 in]
          }
          frame "Macro: Exit" {
            # "Exit Macro\n(This is called once, when the VI exits)"
            n96 = Unbundle By Name(w292) -> ("Core.Close Panel on Exit?"=w302:bool)
            n97 = Select(t="UI: Front Panel State >> Close", s=w302, f="") -> (s? t:f=w299:string)
            n98 = call <vilib>:"Add State(s) to Queue__jki_lib_state_machine.vi"("State(s) in Front (\"\")"="Data: Cleanup\nEvents: Unregister\nProcess: Self Terminate", "State(s) in (\"\")"="Process: Sync", "State(s) at Back (\"\")"="Exit") -> ("States Out"=w294:string)  [unwired: 12 in]
            n99 = call <vilib>:"Add State(s) to Queue__jki_lib_state_machine.vi"("State(s) in Front (\"\")"="Action: Close\nMacro: Write UI Config", "State(s) in (\"\")"=w299, "State(s) at Back (\"\")"=w294) -> ("States Out"=w298:string)  [unwired: 12 in]
            n100 = call <vilib>:"Add State(s) to Queue__jki_lib_state_machine.vi"("State(s) in Front (\"\")"=w298, "State(s) in (\"\")"=w305) -> ("States Out"=w304:string)  [unwired: 13 in]
          }
          frame "---------- Process ----------" {
            # "Template Separator\n(You can make a copy of, or modify, this frame)"
            n101 = call <vilib>:"Add State(s) to Queue__jki_lib_state_machine.vi"("State(s) in (\"\")"=w310) -> ("States Out"=w309:string)  [unwired: 14 in]
          }
          frame "Process: Sync" {
            n102 = Unbundle By Name(w318) -> ("Instrument UI"=w314:refnum<class "Instrument UI.Framework-Template.lvclass">)
            n103 = call <vilib>:"WaitOnProcessSync.vi"("error in (no error)"=w313, "SMO"=w314) -> ("error out"=w312:errorcluster, "Don't run?"=w317:bool)  [unwired: 7 in, 1 out]
            n104 = Select(t="Data: Cleanup\nEvents: Unregister\nExit", s=w317, f="") -> (s? t:f=w311:string)
            n105 = call <vilib>:"Add State(s) to Queue__jki_lib_state_machine.vi"("State(s) in Front (\"\")"=w311, "State(s) in (\"\")"=w321) -> ("States Out"=w320:string)  [unwired: 13 in]
          }
          frame "Process: Self Terminate" {
            n106 = Unbundle By Name(w323) -> ("Instrument UI"=w322:refnum<class "Instrument UI.Framework-Template.lvclass">)
            n107 = call <vilib>:"SelfTerminate.vi"("error in (no error)"=w325, "SMO in"=w322) -> ("error out"=w324:errorcluster)  [unwired: 8 in, 1 out]
            n108 = call <vilib>:"Add State(s) to Queue__jki_lib_state_machine.vi"("State(s) in (\"\")"=w328) -> ("States Out"=w327:string)  [unwired: 14 in]
          }
          frame "---------- Events ----------" {
            # "Template Separator\n(You can make a copy of, or modify, this frame)"
            n109 = call <vilib>:"Add State(s) to Queue__jki_lib_state_machine.vi"("State(s) in (\"\")"=w333) -> ("States Out"=w332:string)  [unwired: 14 in]
          }
          frame "Events: Register" {
            # "Expand to add\nmore events"
            # "Base Class Protected Events"
            n110 = Unbundle By Name(w344) -> ("Instrument UI"=w335:refnum<class "Instrument UI.Framework-Template.lvclass">, "Instrument"=w334:refnum<class "Instrument.Framework-Template.lvclass">)
            n111 = call <vilib>:"GetProtectedEvents.vi"("SMO"=w335) -> ("error out"=w338:errorcluster, "SMO Protected Events"=w342:T9)  [unwired: 8 in, 1 out]
            n112 = call "Instrument.GetPublicEvents.vi"("Instrument"=w334) -> ("error out"=w336:errorcluster, "Instrument Public Events"=w337:T10)  [unwired: 8 in, 1 out]
            n113 = register-events(w342, w337) -> (reference out=w343:refnum<event-registration>, error out=w340:errorcluster)  [unwired: 2 in]
            n114 = Merge Errors(w336, w341, w340, w338) -> (w339:errorcluster)
            n115 = call <vilib>:"Add State(s) to Queue__jki_lib_state_machine.vi"("State(s) in (\"\")"=w346) -> ("States Out"=w345:string)  [unwired: 14 in]
          }
          frame "Events: Unregister" {
            n116 = Unregister For Events(event registration refnum=w349, error in=w348) -> (error out=w347:errorcluster)
            n117 = call <vilib>:"Add State(s) to Queue__jki_lib_state_machine.vi"("State(s) in (\"\")"=w352) -> ("States Out"=w351:string)  [unwired: 14 in]
          }
          frame "---------- Configuration ----------" {
            # "Do not put any code in this frame.\n(It is a separator no-op. You can make a copy of this frame to create a new UI frame)"
            n118 = call <vilib>:"Add State(s) to Queue__jki_lib_state_machine.vi"("State(s) in (\"\")"=w357) -> ("States Out"=w356:string)  [unwired: 14 in]
          }
          frame "Configuration: Initialize" {
            # "Do not put any code in this frame.\n(It is a separator no-op. You can make a copy of this frame to create a new UI frame)"
            n119 = Unbundle By Name(w365) -> ("Configuration"=w363:refnum<class "Configuration.lvclass">, "Instrument"=w364:refnum<class "Instrument.Framework-Template.lvclass">)
            n120 = call <vilib>:"GetName.vi"("error in (no error)"=w367, "SMO"=w364) -> ("error out"=w366:errorcluster, "Name"=w368:string)  [unwired: 6 in, 2 out]
            n121 = call "Default Path.vi"("error in (no error)"=w366, "Folder Name [Application Name]"=w368, "Configuration in"=w363) -> ("error out"=w359:errorcluster, "Configuration out"=w362:refnum<class "Configuration.lvclass">)  [unwired: 7 in]
            n122 = call "Write Section.vi"("error in (no error)"=w359, "Section"="UI", "Configuration in"=w362) -> ("error out"=w358:errorcluster, "Configuration out"=w361:refnum<class "Configuration.lvclass">)  [unwired: 7 in]
            n123 = Bundle By Name(cluster=w365, "Configuration"=w361) -> (w369:T7)
            n124 = call <vilib>:"Add State(s) to Queue__jki_lib_state_machine.vi"("State(s) in (\"\")"=w372) -> ("States Out"=w371:string)  [unwired: 14 in]
          }
          frame "Configuration: Write UI Config File" {
            # "Do not put any code in this frame.\n(It is a separator no-op. You can make a copy of this frame to create a new Data frame)"
            n125 = Unbundle By Name(w377) -> ("Configuration"=w374:refnum<class "Configuration.lvclass">, "UI Cluster"=w376:T6)
            n126 = call "Write Configuration.vi"("error in (no error)"=w373, "Variant"=w376, "Configuration in"=w374) -> ("error out"=w375:errorcluster)  [unwired: 7 in, 1 out]
            n127 = call <vilib>:"Add State(s) to Queue__jki_lib_state_machine.vi"("State(s) in (\"\")"=w380) -> ("States Out"=w379:string)  [unwired: 14 in]
          }
          frame "Configuration: Read UI Config File" {
            # "Do not put any code in this frame.\n(It is a separator no-op. You can make a copy of this frame to create a new UI frame)"
            n128 = Unbundle By Name(w383) -> ("UI Cluster"=w386:T6, "Configuration"=w389:refnum<class "Configuration.lvclass">)
            n129 = call "Read Configuration.vi"("INI Fomatted Cluster Type"=w386, "error in (no error)"=w385, "Configuration in"=w389) -> ("error out"=w388:errorcluster, "Configuration"=w387:variant)  [unwired: 6 in, 1 out]
            n130 = Variant To Data(error in=w388, type=w386, Variant=w387) -> (data=w382:T6, error out=w384:errorcluster)
            n131 = Bundle By Name(cluster=w383, "UI Cluster"=w382) -> (w381:T7)
            n132 = call <vilib>:"Add State(s) to Queue__jki_lib_state_machine.vi"("State(s) in (\"\")"=w392) -> ("States Out"=w391:string)  [unwired: 14 in]
          }
          frame "---------- Action ----------" {
            n133 = Unbundle By Name(w395) -> ("Instrument UI"=w393:refnum<class "Instrument UI.Framework-Template.lvclass">)
            n134 = Bundle By Name(cluster=w395, "Instrument UI"=w393) -> (w394:T7)
            n135 = call <vilib>:"Add State(s) to Queue__jki_lib_state_machine.vi"("State(s) in (\"\")"=w399) -> ("States Out"=w398:string)  [unwired: 14 in]
          }
          frame "Action: Notify UI Closed" {
            # "Notify that the UI has been closed"
            n136 = Unbundle By Name(w400) -> ("Instrument UI"=w403:refnum<class "Instrument UI.Framework-Template.lvclass">)
            n137 = call <vilib>:"Hide.vi"("error in (no error)"=w402, "SMO.UI"=w403) -> ("error out"=w401:errorcluster)  [unwired: 8 in, 1 out]
            n138 = call <vilib>:"Add State(s) to Queue__jki_lib_state_machine.vi"("State(s) in (\"\")"=w406) -> ("States Out"=w405:string)  [unwired: 14 in]
          }
          frame "Action: getAll" {
            n139 = Unbundle By Name(w410) -> ("getAll"=w408:T5, "Instrument"=w413:refnum<class "Instrument.Framework-Template.lvclass">)
            n140 = call "GET ALL.vim"("type"=w408, "error in (no error)"=w411, "Instrument in"=w413) -> ("error out"=w415:errorcluster, "getAll"=w407:T5, "Instrument out"=w409:refnum<class "Instrument.Framework-Template.lvclass">)  [unwired: 6 in]
            n141 = Bundle By Name(cluster=w410, "Instrument"=w409, "getAll"=w407) -> (w412:T7)
            n142 = call <vilib>:"Add State(s) to Queue__jki_lib_state_machine.vi"("State(s) in Front (\"\")"="" ("State(s) in Front (\"\")"), "State(s) in (\"\")"=w418) -> ("States Out"=w417:string)  [unwired: 13 in]
          }
          frame "Action: Open" {
            n143 = Unbundle By Name(w425) -> ("Instrument"=w423:refnum<class "Instrument.Framework-Template.lvclass">)
            n144 = call "Write Client Type.vi"("error in (no error)"=w420, "Client Type"=Client_Type--Enum."Local", "Instrument in"=w423) -> ("error out"=w421:errorcluster, "Instrument out"=w422:refnum<class "Instrument.Framework-Template.lvclass">)  [unwired: 7 in]
            n145 = call-dynamic "Open.vi"("error in (no error)"=w421, "Instrument.Template in"=w422) -> ("error out"=w428:errorcluster, "Instrument.Template out"=w424:refnum<class "Instrument.Framework-Template.lvclass">)  [unwired: 8 in]
            n146 = Bundle By Name(cluster=w425, "Instrument"=w424) -> (w426:T7)
            n147 = call <vilib>:"Add State(s) to Queue__jki_lib_state_machine.vi"("State(s) in Front (\"\")"="" ("State(s) in Front (\"\")"), "State(s) in (\"\")"=w431) -> ("States Out"=w430:string)  [unwired: 13 in]
          }
          frame "Action: Close" {
            n148 = Unbundle By Name(w433) -> ("Instrument"=w436:refnum<class "Instrument.Framework-Template.lvclass">)
            n149 = call-dynamic "Close.vi"("error in (no error)"=w434, "Instrument.Template in"=w436) -> ("error out"=w438:errorcluster, "Instrument.Template out"=w432:refnum<class "Instrument.Framework-Template.lvclass">)  [unwired: 8 in]
            n150 = Bundle By Name(cluster=w433, "Instrument"=w432) -> (w435:T7)
            n151 = call <vilib>:"Add State(s) to Queue__jki_lib_state_machine.vi"("State(s) in Front (\"\")"="" ("State(s) in Front (\"\")"), "State(s) in (\"\")"=w441) -> ("States Out"=w440:string)  [unwired: 13 in]
          }
          frame "Action: setConfiguration" {
            n152 = Unbundle By Name(w444) -> ("Instrument"=w447:refnum<class "Instrument.Framework-Template.lvclass">, "Config Cluster"=w442:T4)
            n153 = call "SET CONFIG.vim"("error in (no error)"=w445, "Configuration"=w442, "Instrument in"=w447) -> ("error out"=w449:errorcluster, "Instrument out"=w443:refnum<class "Instrument.Framework-Template.lvclass">)  [unwired: 7 in]
            n154 = Bundle By Name(cluster=w444, "Instrument"=w443) -> (w446:T7)
            n155 = call <vilib>:"Add State(s) to Queue__jki_lib_state_machine.vi"("State(s) in Front (\"\")"="" ("State(s) in Front (\"\")"), "State(s) in (\"\")"=w452) -> ("States Out"=w451:string)  [unwired: 13 in]
          }
        }
      }
    }
    frame Error {
    }
  }
  n156 = call-parent "Process.vi"("error in"=w5, "Instrument UI in"=w4) -> ("error out"=w2:errorcluster, "Instrument UI out"=→"Example Instrument UI out":refnum<class "Instrument UI.Framework-Template.lvclass">)  [unwired: 8 in]
  n157 = Merge Errors(w2, w1) -> (→"error out":errorcluster)
